vi "set_voltage.vi"(4 "lower limit":dbl format="%#_13g", 6 "upper limit":dbl=5.0 format="%#_13g", 8 "error in (no error)":errorcluster, 10 "value":dbl, 11 "VISA resource name":refnum<visa-resource-name>="Tenma") -> (0 "error out":errorcluster, 2 "value_out":dbl, 3 "VISA resource name out":refnum<visa-resource-name>)   [LabVIEW 2017, in "tenma.lvlib"]
doc: "<B>Laser Goto with FCU</B> VI tunes laser to the position <B>Wavenumber (1/cm)</B>. FCU1 is adjusted accordingly."
uses:
  <vilib>/Instr/_visa.llb/VISA Configure Serial Port (Instr).vi
  tenma.lvlib
panel:
  out "output string":string
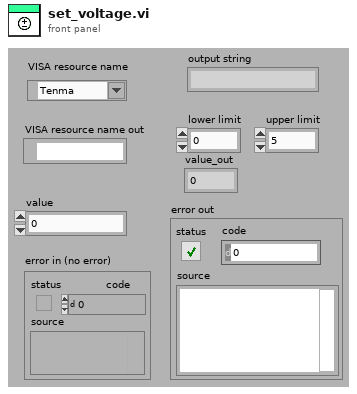
[diagram p1: front panel]
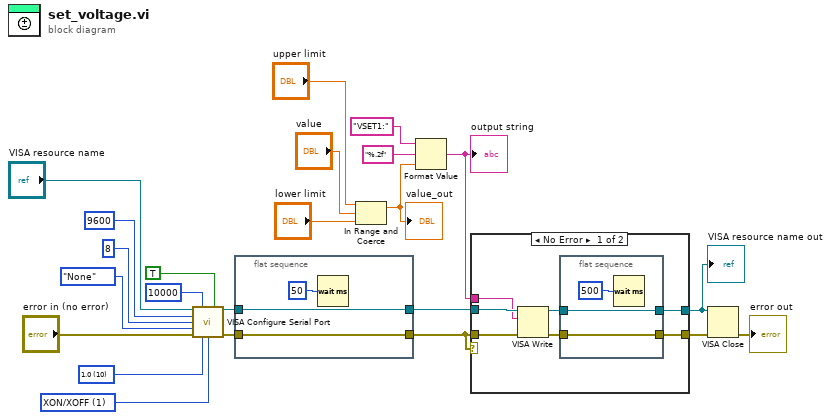
[diagram p0: block diagram]
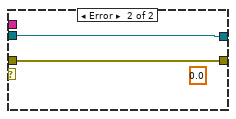
[diagram p2: hidden frame]
diagram:
  w9 = u16 1 items=["None", "XON/XOFF", "RTS/CTS", "XON/XOFF & RTS/CTS", "DTR/DSR", "XON/XOFF & DTR/DSR"] ("flow control (0:none)")
  w10 = u16 10 items=["1.0"=10, "1.5"=15, "2.0"=20] ("stop bits (10: 1 bit)")
  n1 = call-poly "VISA Configure Serial Port"("VISA resource name"="VISA resource name", "timeout (10sec)"=u32 10000, "Enable Termination\nChar (T)"=TRUE ("Enable Termination\nChar (T)"), "baud rate (9600)"=u32 9600, "data bits (8)"=u16 8, "parity (0:none)"=enum16{"None", "Odd", "Even", "Mark", "Space"}."None", "error in (no error)"="error in (no error)", "stop bits (10: 1 bit)"=w10, "flow control (0:none)"=w9) -> ("VISA resource name out"=w15:refnum<visa-resource-name>, "error out"=w13:errorcluster)  [unwired: 5 in]
  n2 = flat-sequence {
    tunnel: w15 -> [w26]
    tunnel: [w26] -> w14
    tunnel: w13 -> [w25]
    tunnel: [w25] -> w12
    frame #0 {
      n3 = Wait (ms)(milliseconds to wait=u32 50) -> ()  [unwired: 1 out]
    }
  }
  n4 = In Range and Coerce(upper limit="upper limit", x="value", lower limit="lower limit") -> (coerced(x)=w2:dbl)  [unwired: 1 out]
  "value_out" <- w2
  n5 = Format Value(string ("")="VSET1:" ("write"), format string="%.2f", value (0)=w2) -> (output string=w1:string)
  "output string" <- w1
  n6 = case shown="No Error" w12 {
    tunnel: w12 -> [w31 w38]
    tunnel: w14 -> [w30 w37]
    tunnel: [w29 w38] -> w19
    tunnel: [w28 w37] -> w8
    tunnel: w1 -> [w27 _]
    frame No Error {
      n7 = VISA Write(VISA resource name=w30, write buffer=w27, error in (no error)=w31) -> (VISA resource name out=w33:refnum<visa-resource-name>, error out=w32:errorcluster)  [unwired: 1 out]
      n8 = flat-sequence {
        tunnel: w33 -> [w36]
        tunnel: [w36] -> w28
        tunnel: w32 -> [w35]
        tunnel: [w35] -> w29
        frame #0 {
          n9 = Wait (ms)(milliseconds to wait=u32 500) -> ()  [unwired: 1 out]
        }
      }
    }
    frame Error {
      (unwired) 0.0
    }
  }
  "VISA resource name out" <- w8
  n10 = VISA Close(VISA resource name=w8, error in (no error)=w19) -> (error out=→"error out":errorcluster)
